vi "PI_Scanrange_limit.vi"(8 "Input Cluster":T6, 10 "Enum":enum32{"Stage", "Mirror"}(ring)) -> (0 "Output Cluster":T6)   [LabVIEW 2009]
uses:
  atmcd32d.llb/AcquisitionMode_mode typedef.ctl
  atmcd32d.llb/ReadMode_mode typedef.ctl
  atmcd32d.llb/TriggerMode_mode typedef.ctl
  atmcd32d.llb/Shutter_type typedef.ctl
  atmcd32d.llb/Shutter_mode typedef.ctl
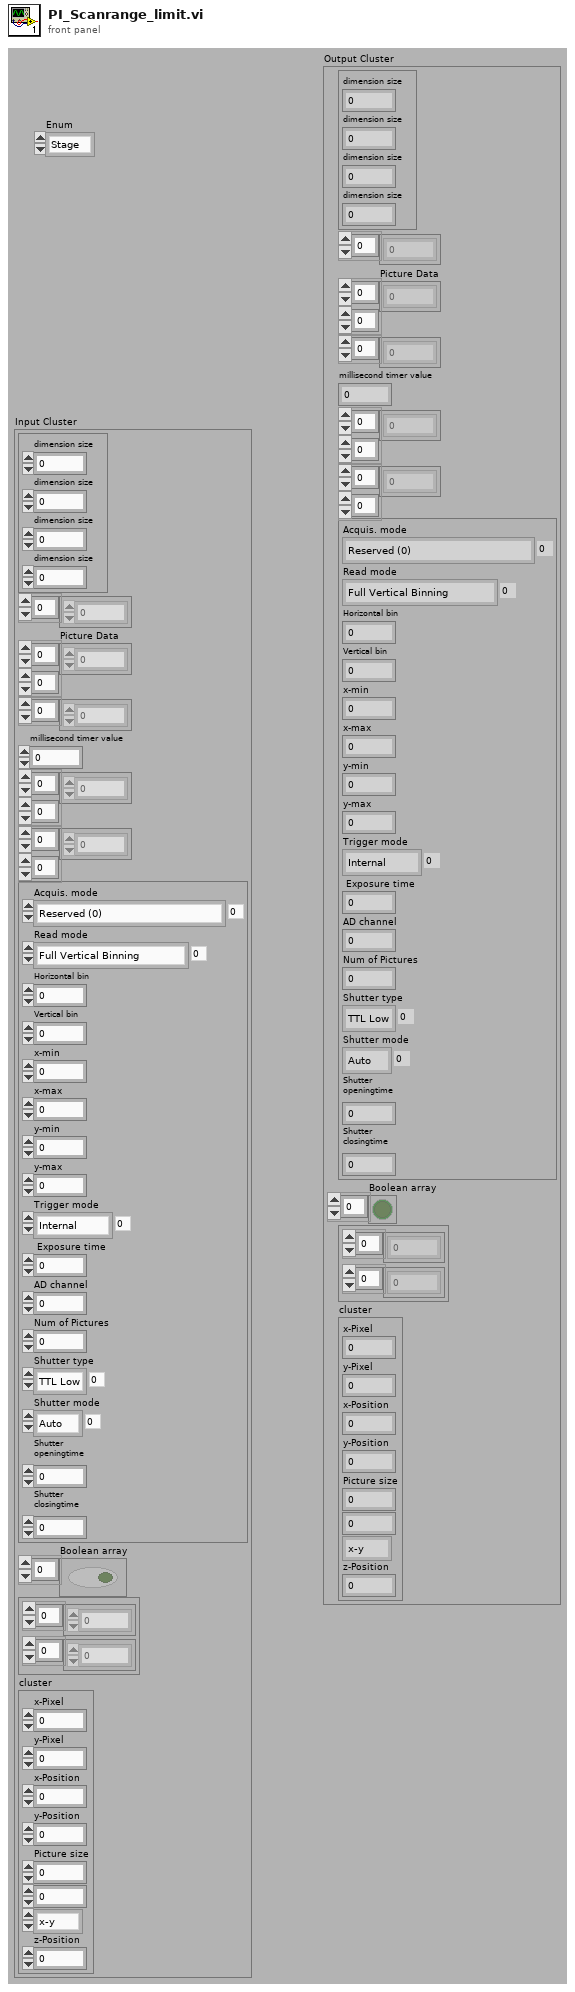
[diagram p1: front panel]
types:
  T1 = typedef "AcquisitionMode_mode typedef.ctl" = enum16{"Reserved (0)", "Single Scan", "Accumulate", "Kinetics", "Fast Kinetics", "Run Till Abort", "Reserved (6)", "Reserved (7)", "Reserved (8)", "Time Delayed Integration"}
  T2 = typedef "ReadMode_mode typedef.ctl" = enum16{"Full Vertical Binning", "Multi-Track", "Random-Track", "Single-Track", "Image"}
  T3 = typedef "TriggerMode_mode typedef.ctl" = enum16{"Internal", "External", "N/A (2)", "N/A (3)", "N/A (4)", "N/A (5)", "External Start"}
  T4 = typedef "Shutter_type typedef.ctl" = enum16{"TTL Low", "TTL High"}
  T5 = typedef "Shutter_mode typedef.ctl" = enum16{"Auto", "Open", "Close"}
  T6 = cluster{cluster{"dimension size":i32, "dimension size":i32, "dimension size":i32, "dimension size":i32}, i32[], "Picture Data":dbl[][], u32[], "millisecond timer value":u32, dbl[][], i32[][], cluster{"Acquis. mode":T1, "Read mode":T2, "Horizontal bin":i32, "Vertical bin":i32, "x-min":i32, "x-max":i32, "y-min":i32, "y-max":i32, "Trigger mode":T3, " Exposure time":sgl, "AD channel":i32, "Num of Pictures":i32, "Shutter type":T4, "Shutter mode":T5, "Shutter\nopeningtime":i32, "Shutter\nclosingtime":i32}, "Boolean array":bool[], cluster{dbl[], dbl[]}, "cluster":cluster{"x-Pixel":u16, "y-Pixel":u16, "x-Position":dbl, "y-Position":dbl, "Picture size":dbl, dbl, enum32{"x-y", "x-z", "y-z"}, "z-Position":dbl}}
  T7 = cluster{"x-Pixel":u16, "y-Pixel":u16, "x-Position":dbl, "y-Position":dbl, "Picture size":dbl, dbl, enum32{"x-y", "x-z", "y-z"}, "z-Position":dbl}
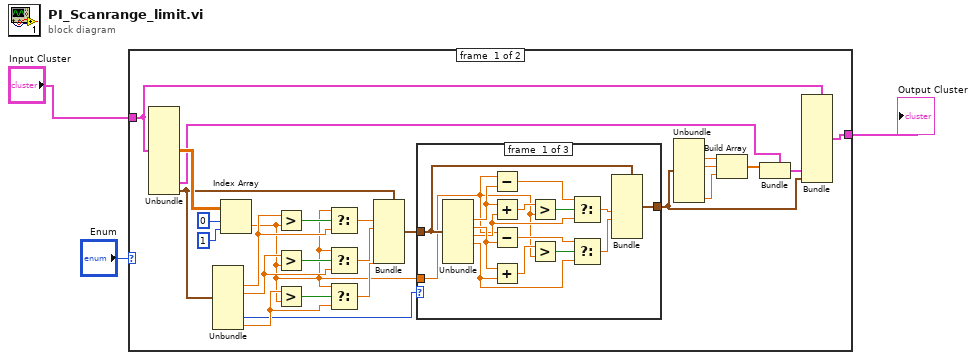
[diagram p0: block diagram]
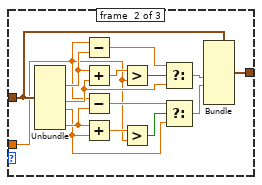
[diagram p2: hidden frame]
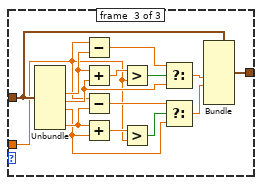
[diagram p3: hidden frame]
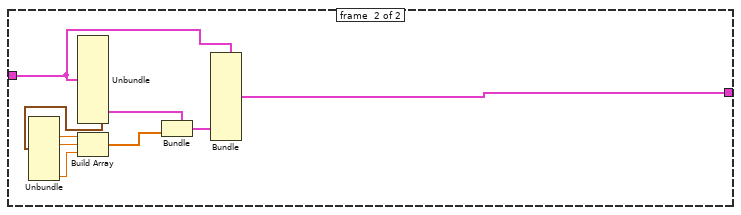
[diagram p4: hidden frame]
diagram:
  n1 = case shown="\"Stage\", Default" "Enum" {
    tunnel: "Input Cluster" -> [w10 w77]
    tunnel: [w8 w75] -> w3
    frame #0 {
      n2 = Unbundle(w10) -> (w28:dbl[][], w15:cluster{dbl[], dbl[]}, "cluster"=w5:T7)  [unwired: 8 out]
      n3 = Unbundle(w5) -> ("x-Position"=w24:dbl, "y-Position"=w21:dbl, w17:enum32{"x-y", "x-z", "y-z"}, "z-Position"=w20:dbl)  [unwired: 4 out]
      n4 = Index Array(array=w28, index (row)=0, index (col)=1 ("disabled index (col)")) -> (element=w6:dbl)
      n5 = Greater?(x=w24, y=w6) -> (0:w25:bool)
      n6 = Greater?(x=w21, y=w6) -> (0:w23:bool)
      n7 = Greater?(x=w20, y=w6) -> (0:w22:bool)
      n8 = Select(t=w6, s=w25, f=w24) -> (s? t:f=w19:dbl)
      n9 = Select(t=w6, s=w23, f=w21) -> (s? t:f=w18:dbl)
      n10 = Select(t=w6, s=w22, f=w20) -> (s? t:f=w7:dbl)
      n11 = Bundle(cluster=w5, "x-Position"=w19, "y-Position"=w18, "z-Position"=w7) -> (w16:T7)  [unwired: 5 out]
      n12 = case shown="\"x-y\", Default" w17 {
        tunnel: w16 -> [w33 w48 w70]
        tunnel: w6 -> [w29 w44 w59]
        tunnel: [w32 w47 w63] -> w4
        frame #0 {
          n13 = Unbundle(w33) -> ("x-Position"=w30:dbl, "y-Position"=w36:dbl, "Picture size"=w35:dbl, w31:dbl)  [unwired: 4 out]
          n14 = Subtract(x=w29, y=w30) -> (x-y=w41:dbl)
          n15 = Add(x=w30, y=w35) -> (x+y=w43:dbl)
          n16 = Subtract(x=w29, y=w36) -> (x-y=w37:dbl)
          n17 = Add(x=w36, y=w31) -> (x+y=w39:dbl)
          n18 = Greater?(x=w43, y=w29) -> (0:w42:bool)
          n19 = Greater?(x=w39, y=w29) -> (0:w38:bool)
          n20 = Select(t=w41, s=w42, f=w35) -> (s? t:f=w40:dbl)
          n21 = Select(t=w37, s=w38, f=w31) -> (s? t:f=w34:dbl)
          n22 = Bundle(cluster=w33, "Picture size"=w40, w34) -> (w32:T7)  [unwired: 6 out]
        }
        frame #1 {
          n23 = Unbundle(w48) -> ("x-Position"=w56:dbl, "Picture size"=w50:dbl, w45:dbl, "z-Position"=w46:dbl)  [unwired: 4 out]
          n24 = Subtract(x=w44, y=w56) -> (x-y=w55:dbl)
          n25 = Add(x=w56, y=w50) -> (x+y=w58:dbl)
          n26 = Subtract(x=w44, y=w46) -> (x-y=w51:dbl)
          n27 = Add(x=w46, y=w45) -> (x+y=w53:dbl)
          n28 = Greater?(x=w58, y=w44) -> (0:w57:bool)
          n29 = Greater?(x=w53, y=w44) -> (0:w52:bool)
          n30 = Select(t=w55, s=w57, f=w50) -> (s? t:f=w54:dbl)
          n31 = Select(t=w51, s=w52, f=w45) -> (s? t:f=w49:dbl)
          n32 = Bundle(cluster=w48, "Picture size"=w54, w49) -> (w47:T7)  [unwired: 6 out]
        }
        frame #2 {
          n33 = Unbundle(w70) -> ("y-Position"=w61:dbl, "Picture size"=w65:dbl, w60:dbl, "z-Position"=w62:dbl)  [unwired: 4 out]
          n34 = Subtract(x=w59, y=w61) -> (x-y=w71:dbl)
          n35 = Add(x=w61, y=w65) -> (x+y=w73:dbl)
          n36 = Subtract(x=w59, y=w62) -> (x-y=w66:dbl)
          n37 = Add(x=w62, y=w60) -> (x+y=w68:dbl)
          n38 = Greater?(x=w73, y=w59) -> (0:w72:bool)
          n39 = Greater?(x=w68, y=w59) -> (0:w67:bool)
          n40 = Select(t=w71, s=w72, f=w65) -> (s? t:f=w69:dbl)
          n41 = Select(t=w66, s=w67, f=w60) -> (s? t:f=w64:dbl)
          n42 = Bundle(cluster=w70, "Picture size"=w69, w64) -> (w63:T7)  [unwired: 6 out]
        }
      }
      n43 = Unbundle(w4) -> ("x-Position"=w13:dbl, "y-Position"=w12:dbl, "z-Position"=w11:dbl)  [unwired: 5 out]
      n44 = Build Array(w13, w12, w11) -> (w14:dbl[])
      n45 = Bundle(cluster=w15, w14) -> (w9:cluster{dbl[], dbl[]})  [unwired: 1 out]
      n46 = Bundle(cluster=w10, w9, "cluster"=w4) -> (w8:T6)  [unwired: 9 out]
    }
    frame #1 {
      n47 = Unbundle(w77) -> (w79:cluster{dbl[], dbl[]}, "cluster"=w74:T7)  [unwired: 9 out]
      n48 = Unbundle(w74) -> ("x-Position"=w82:dbl, "y-Position"=w81:dbl, "z-Position"=w80:dbl)  [unwired: 5 out]
      n49 = Build Array(w82, w81, w80) -> (w78:dbl[])
      n50 = Bundle(cluster=w79, w78) -> (w76:cluster{dbl[], dbl[]})  [unwired: 1 out]
      n51 = Bundle(cluster=w77, w76) -> (w75:T6)  [unwired: 10 out]
    }
  }
  "Output Cluster" <- w3
